vi "Read.vi"(8 "error in (no error)":errorcluster, 11 "Accelerometer Ref In":T1) -> (0 "error out":errorcluster, 2 "Values":dbl[](array[numeric]), 3 "Accelerometer Ref Out":T1)   [LabVIEW 2021, in "Accelerometer.lvlib"]
doc: "Reads acceleration values from the onboard accelerometer. You must open and configure accelerometer channels before reading values from the accelerometer channels."
uses:
  <vilib>/myRIO/Instrument Drivers/Onboard Devices/Accelerometer/Accelerometer.lvlib
  <vilib>/myRIO/Instrument Drivers/Onboard Devices/Accelerometer/typedefs/Accelerometer Reference.ctl
  <vilib>/myRIO/Common/Instrument Driver Framework/Utilities/typedefs/myRIO Generic Hardware Reference.ctl
  <vilib>/myRIO/Common/Instrument Driver Framework/Utilities/typedefs/Hardware Version Enum.ctl
  <vilib>/myRIO/Common/Instrument Driver Framework/Utilities/typedefs/myRIO v1.0 Reference.ctl
  <vilib>/myRIO/Common/Instrument Driver Framework/Utilities/typedefs/Generic FPGA Reference.ctl
  <vilib>/myRIO/Common/Instrument Driver Framework/myRIO v1.0/Accelerometer/typedefs/Accelerometer Channels List.ctl
  <vilib>/myRIO/Common/Instrument Driver Framework/myRIO v1.0/Accelerometer/typedefs/Accelerometer Channels Enum.ctl
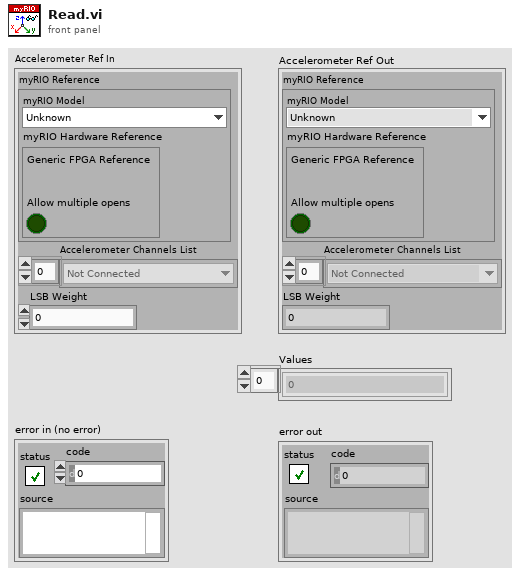
[diagram p1: front panel]
types:
  T1 = typedef "Accelerometer.lvlib/Accelerometer Reference.ctl" = cluster{"myRIO Reference":T2, "Accelerometer Channels List":T6, "LSB Weight":dbl}
  T2 = typedef "myRIO Generic Hardware Reference.ctl" = cluster{"myRIO Model":T3, "myRIO Hardware Reference":T4}
  T3 = typedef "Hardware Version Enum.ctl" = enum16{"Unknown", "myRIO-1900", "myRIO-1950", "roboRIO", "NI ELVIS RIO CM", "ELVIS III"}
  T4 = typedef "myRIO v1.0 Reference.ctl" = cluster{"Generic FPGA Reference":T5, "Allow multiple opens":bool}
  T5 = typedef "Generic FPGA Reference.ctl" = refnum<k20>
  T6 = typedef "Accelerometer Channels List.ctl" = T7[]
  T7 = typedef "Accelerometer Channels Enum.ctl" = enum16{"Not Connected", "X-Axis", "Y-Axis", "Z-Axis"}
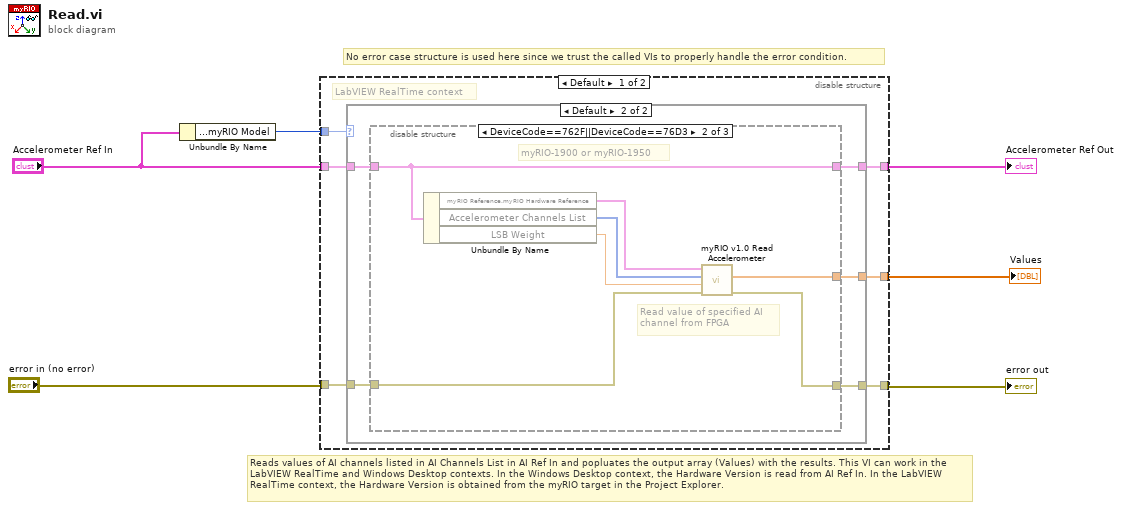
[diagram p0: block diagram]
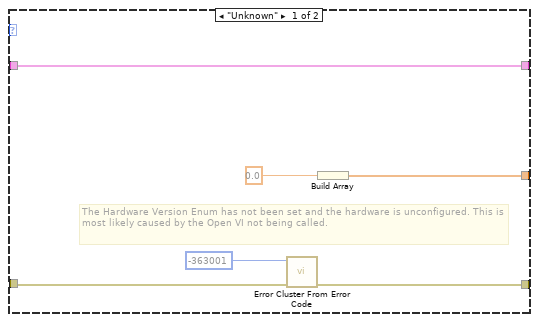
[diagram p2: hidden frame]
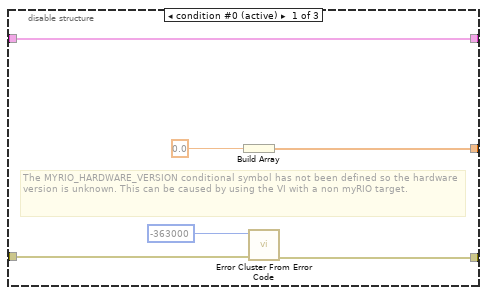
[diagram p3: hidden frame]
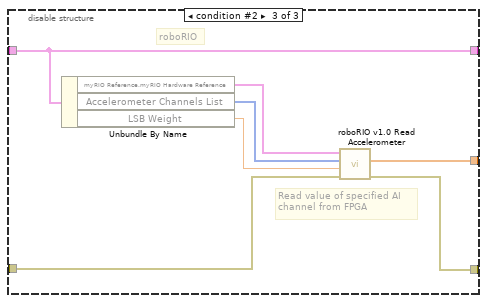
[diagram p4: hidden frame]
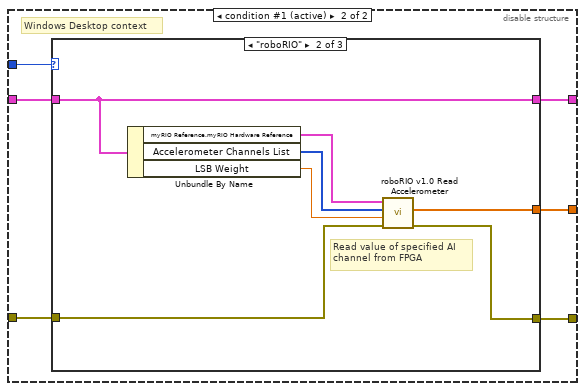
[diagram p5: hidden frame]
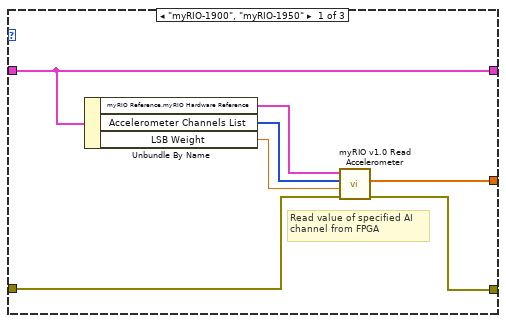
[diagram p6: hidden frame]
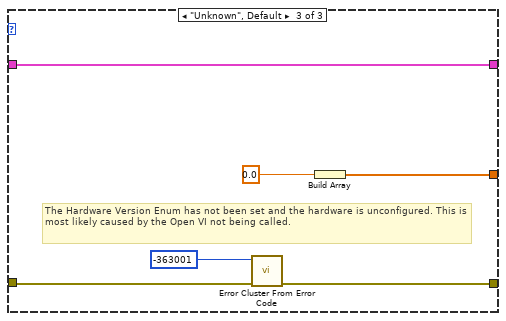
[diagram p7: hidden frame]
diagram:
  # "No error case structure is used here since we trust the called VIs to properly handle the error condition."
  # "Reads values of AI channels listed in AI Channels List in AI Ref In and popluates the output array (Values) with the results. This VI can work in the LabVIEW RealTime and Windows Desktop contexts. In the Windows Desktop context, the Hardware Version is read from AI Ref In. In the LabVIEW RealTime context, the Hardware Version is obtained from the myRIO target in the Project Explorer."
  n1 = Unbundle By Name("Accelerometer Ref In") -> ("myRIO Reference.myRIO Model"=w1:T3)
  n2 = disable-structure shown="Default" {
    disable-tunnel: [w12 w49] -> w3
    disable-tunnel: "Accelerometer Ref In" -> [w11 w46]
    disable-tunnel: "error in (no error)" -> [w10 w48]
    disable-tunnel: [w9 w47] -> w4
    disable-tunnel: [w8 w45] -> w2
    disable-tunnel: w1 -> [w7 w44]
    frame condition #0 {
      # "LabVIEW RealTime context"
      n3 = case shown="Default" w7 {
        tunnel: [w15 w23] -> w12
        tunnel: w11 -> [w13 w22]
        tunnel: w10 -> [w16 w21]
        tunnel: [w13 w20] -> w9
        tunnel: [w14 w19] -> w8
        frame "Unknown" {
          # "The Hardware Version Enum has not been set and the hardware is unconfigured. This is most likely caused by the Open VI not being called."
          n4 = call <vilib>:"Error Cluster From Error Code.vi"("error in (no error)"=w16, "error code (0)"=-363001) -> ("error out"=w15:errorcluster)  [unwired: 7 in]
          n5 = Build Array(0.0 ("dbl Scaled Value")) -> (w14:dbl[])
        }
        frame Default {
          n6 = disable-structure shown="DeviceCode==762F||DeviceCode==76D3" {
            disable-tunnel: w22 -> [w26 w35 w42]
            disable-tunnel: [w29 w31 w38] -> w23
            disable-tunnel: [w24 w32 w39] -> w19
            disable-tunnel: w21 -> [w27 w34 w41]
            disable-tunnel: [w26 w35 w42] -> w20
            frame condition #0 (active) {
              # "The MYRIO_HARDWARE_VERSION conditional symbol has not been defined so the hardware version is unknown. This can be caused by using the VI with a non myRIO target."
              n7 = Build Array(0.0 ("dbl Scaled Value")) -> (w24:dbl[])
              n8 = call <vilib>:"Error Cluster From Error Code.vi"("error in (no error)"=w27, "error code (0)"=-363000) -> ("error out"=w29:errorcluster)  [unwired: 7 in]
            }
            frame condition #1 {
              # "myRIO-1900 or myRIO-1950"
              # "Read value of specified AI \nchannel from FPGA"
              n9 = Unbundle By Name(w35) -> ("myRIO Reference.myRIO Hardware Reference"=w36:T4, "Accelerometer Channels List"=w33:T6, "LSB Weight"=w30:dbl)
              n10 = call <vilib>:"myRIO v1.0 Read Accelerometer.vi"("error in (no error)"=w34, "LSB Weight (g-force/bit)"=w30, "Channel List"=w33, "myRIO Ref In"=w36) -> ("error out"=w31:errorcluster, "dbl Scaled Value List"=w32:dbl[])  [unwired: 5 in, 1 out]
            }
            frame condition #2 {
              # "roboRIO"
              # "Read value of specified AI \nchannel from FPGA"
              n11 = Unbundle By Name(w42) -> ("myRIO Reference.myRIO Hardware Reference"=w43:T4, "Accelerometer Channels List"=w40:T6, "LSB Weight"=w37:dbl)
              n12 = call <vilib>:"roboRIO v1.0 Read Accelerometer.vi"("error in (no error)"=w41, "LSB Weight (g-force/bit)"=w37, "Channel List"=w40, "myRIO Ref In"=w43) -> ("error out"=w38:errorcluster, "dbl Scaled Value List"=w39:dbl[])  [unwired: 5 in, 1 out]
            }
          }
        }
      }
    }
    frame condition #1 (active) {
      # "Windows Desktop context"
      n13 = case shown="\"roboRIO\"" w44 {
        tunnel: [w52 w59 w69] -> w49
        tunnel: w46 -> [w56 w63 w66]
        tunnel: w48 -> [w53 w60 w67]
        tunnel: [w56 w63 w66] -> w47
        tunnel: [w51 w58 w64] -> w45
        frame "myRIO-1900", "myRIO-1950" {
          # "Read value of specified AI \nchannel from FPGA"
          n14 = Unbundle By Name(w56) -> ("myRIO Reference.myRIO Hardware Reference"=w55:T4, "Accelerometer Channels List"=w54:T6, "LSB Weight"=w50:dbl)
          n15 = call <vilib>:"myRIO v1.0 Read Accelerometer.vi"("error in (no error)"=w53, "LSB Weight (g-force/bit)"=w50, "Channel List"=w54, "myRIO Ref In"=w55) -> ("error out"=w52:errorcluster, "dbl Scaled Value List"=w51:dbl[])  [unwired: 5 in, 1 out]
        }
        frame "roboRIO" {
          # "Read value of specified AI \nchannel from FPGA"
          n16 = Unbundle By Name(w63) -> ("myRIO Reference.myRIO Hardware Reference"=w62:T4, "Accelerometer Channels List"=w61:T6, "LSB Weight"=w57:dbl)
          n17 = call <vilib>:"roboRIO v1.0 Read Accelerometer.vi"("error in (no error)"=w60, "LSB Weight (g-force/bit)"=w57, "Channel List"=w61, "myRIO Ref In"=w62) -> ("error out"=w59:errorcluster, "dbl Scaled Value List"=w58:dbl[])  [unwired: 5 in, 1 out]
        }
        frame "Unknown", Default {
          # "The Hardware Version Enum has not been set and the hardware is unconfigured. This is most likely caused by the Open VI not being called."
          n18 = call <vilib>:"Error Cluster From Error Code.vi"("error in (no error)"=w67, "error code (0)"=-363001) -> ("error out"=w69:errorcluster)  [unwired: 7 in]
          n19 = Build Array(0.0 ("dbl Scaled Value")) -> (w64:dbl[])
        }
      }
    }
  }
  "Accelerometer Ref Out" <- w4
  "error out" <- w3
  "Values" <- w2
